vi "Rebuild from Tree.vi"(8 "error in (no error)":errorcluster, 10 "Tag":string, 11 "Tree Manager in":refnum<class "Tree Manager.lvclass">) -> (0 "error out":errorcluster, 2 "Rebuilt Item":refnum<class "Data Item.lvclass">, 3 "Tree Manager out":refnum<class "Tree Manager.lvclass">)   [LabVIEW 2020, in "VILab.lvlib" / "Tree Manager.lvclass"]
uses:
  Tree Manager.lvclass
  Data Item/Data Item.lvclass
  Tree Manager.lvclass/Tree Manager.ctl
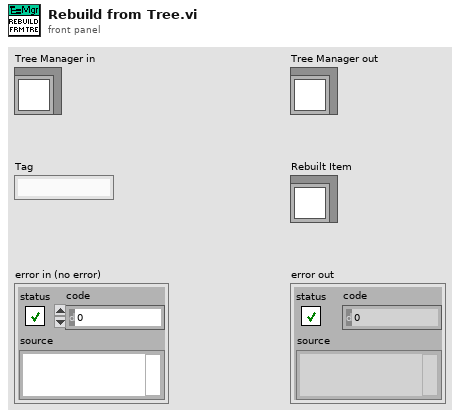
[diagram p1: front panel]
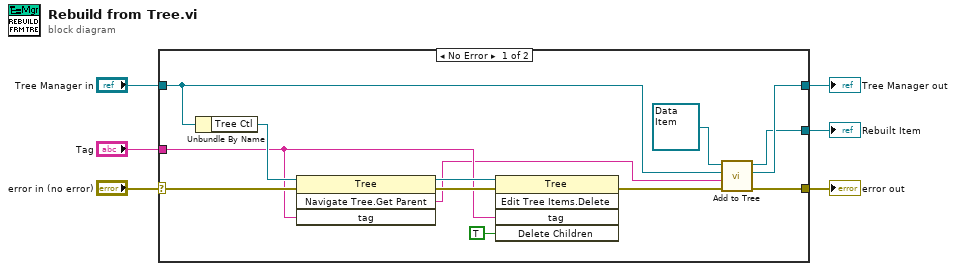
[diagram p0: block diagram]
diagram:
  n1 = case shown="No Error" "error in (no error)" {
    selector: "error in (no error)" -> [w16 w21]
    tunnel: [w12 w21] -> w5
    tunnel: [w13 w20] -> w3
    tunnel: "Tree Manager in" -> [w8 w20]
    tunnel: "Tag" -> [w10 _]
    tunnel: [w7 _] -> w1
    frame No Error {
      n2 = Unbundle By Name(w8) -> ("Tree Ctl"=w17:refnum<vi>)
      n3 = invoke class="Tree" method="Navigate Tree.Get Parent"(reference=w17, error in=w16, "tag"=w10) -> (reference out=w15:refnum<vi>, error out=w14:errorcluster, "Navigate Tree:Get Parent"=w9:string)  [unwired: 1 in, 1 out]
      n4 = invoke on="Delete" class="Tree" method="Edit Tree Items.Delete"(reference=w15, error in=w14, "tag"=w10, "Delete Children"=TRUE ("Delete Children?")) -> (error out=w18:errorcluster)  [unwired: 1 in, 4 out]
      n5 = call-dynamic "Add to Tree.vi"("error in (no error)"=w18, "Parent Tag"=w9, "Tree Manager in"=w8, "Data Item in"=refnum<class "Data Item.lvclass"> refnum) -> ("error out"=w12:errorcluster, "Tree Manager out"=w13:refnum<class "Tree Manager.lvclass">, "Data Item out"=w7:refnum<class "Data Item.lvclass">)  [unwired: 5 in]
    }
    frame Error {
    }
  }
  "error out" <- w5
  "Tree Manager out" <- w3
  "Rebuilt Item" <- w1
